vi "Actor Core.vi"(8 "error in":errorcluster, 11 "Screw in":refnum<class "Screw.lvclass">) -> (0 "error out":errorcluster, 3 "Actor out":refnum<class "Actor.lvclass">)   [LabVIEW 2018, in "Feeder Actor.lvlib" / "Screw.lvclass"]
doc: "(<B>Filename</B>: Actor Framework.lvlib:Actor.lvclass:Actor Core.vi)\n\nReceives messages to the actor, reacts to them, and initiates any error handling that may shut the actor down.\n\nDescendant classes may override this VI to append parallel tasks for the actor to complete while it handles messages. Overrides use the Call Parent Method node."
uses:
  Screw.lvclass
  <vilib>/ActorFramework/Actor/Actor.lvclass
  Screw.lvclass/Screw.ctl
  <vilib>/MGI/Panel Manager/Panel Actor/Panel Actor/Panel Actor.lvclass
panel:
  in  "Screw":u16(ring) items=["0%"=1, "25%"=225, "50%"=450, "75%"=675, "100%"=900]
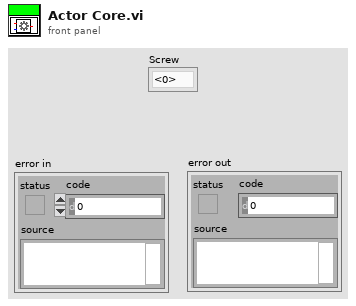
[diagram p1: front panel]
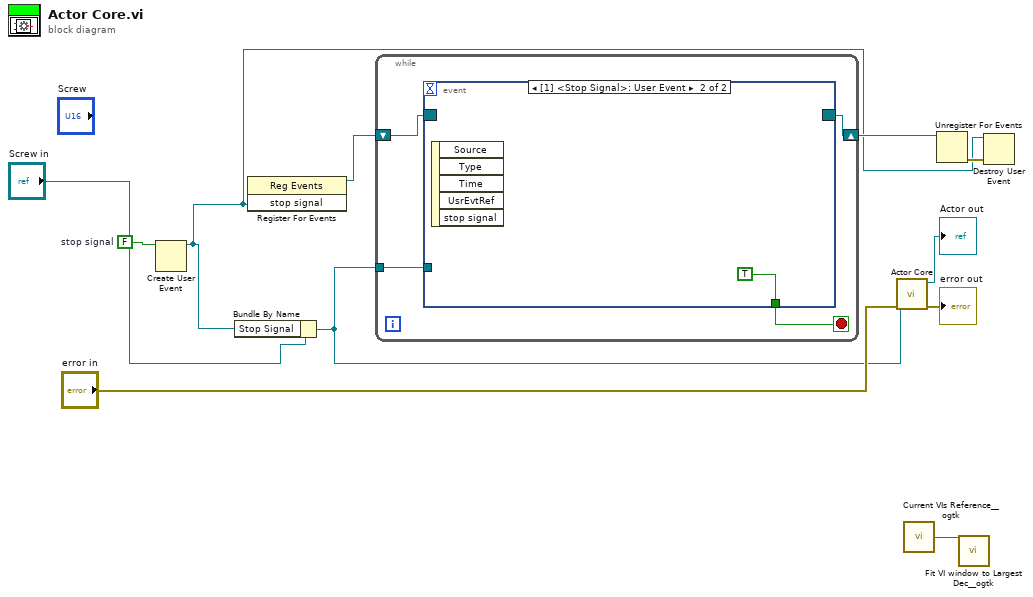
[diagram p0: block diagram]
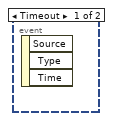
[diagram p2: hidden frame]
diagram:
  w4 = FALSE  # stop signal
  n1 = Create User Event(user event datatype=w4) -> (user event=w3:refnum<user-event>)  [unwired: 1 in, 1 out]
  n2 = Bundle By Name(cluster="Screw in", "Stop Signal"=w3) -> (w1:refnum<class "Screw.lvclass">)
  n3 = register-events(w3) -> (reference out=w7:refnum<event-registration>)  [unwired: 2 in, 1 out]
  n4 = while {
    shift-right: [w13] -> w5
    shift-left: w7 -> [w14]
    tunnel: w1 -> [w12]
    stop <- w15 stop-if-true
    n5 = event shown="[1] <Stop Signal>: User Event" {
      selector: w14 -> [_ _]
      dyn-events: [_ _] -> w13
      timeout: _ -> [_ _]
      tunnel: [_ TRUE] -> w15
      tunnel: w12 -> [_ _]
      event Timeout {
        n6 = event-data() -> ()  [unwired: 1 in, 3 out]
      }
      event User Event {
        n7 = event-data() -> ()  [unwired: 1 in, 5 out]
      }
    }
  }
  n8 = call-parent "Actor Core.vi"("error in"="error in", "Panel Actor in"=w1) -> ("error out"=→"error out":errorcluster, "Actor out"=→"Actor out":refnum<class "Actor.lvclass">)  [unwired: 8 in]
  n9 = call <userlib>:"Current VIs Reference__ogtk.vi"() -> ("Current VI's reference"=w8:refnum<vi>)  [unwired: 5 in]
  n10 = Unregister For Events(event registration refnum=w5) -> (error out=w6:errorcluster)  [unwired: 1 in]
  n11 = call <userlib>:"Fit VI window to Largest Dec__ogtk.vi"("VI Ref (calling VI)"=w8) -> ()  [unwired: 5 in, 2 out]
  n12 = Destroy User Event(user event=w3, error in=w6) -> ()  [unwired: 1 out]
